vi "video.create_free.vi"(8 "error in":errorcluster, 11 "VideoCreateStaging":refnum<class "VideoCreateStaging.lvclass">) -> (0 "error out":errorcluster)   [LabVIEW 2020, in "VideoCreateStaging.lvclass"]
doc: "Releases the handle and its associated resources."
uses:
  VideoCreateStaging.lvclass
  VideoCreateStaging.lvclass/VideoCreateStaging.ctl
  client.lvlib
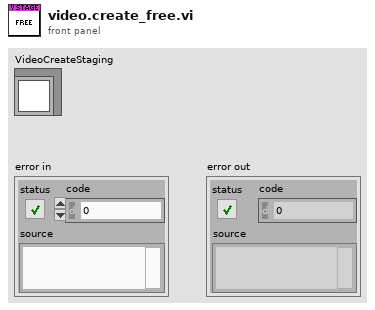
[diagram p1: front panel]
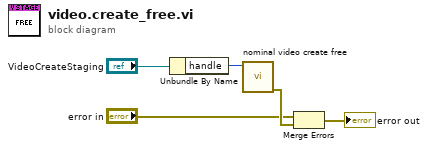
[diagram p0: block diagram]
diagram:
  n1 = Unbundle By Name("VideoCreateStaging") -> ("handle"=w5:i32)
  n2 = call "nominal video create free.vi"("staging"=w5) -> ("error out"=w3:errorcluster)  [unwired: 9 in, 1 out]
  n3 = Merge Errors("error in", w3) -> (→"error out":errorcluster)
